vi "image LPF-cluster.vi"(1 "image lpf":cluster{"cutoff ":dbl, "lpf":bool, "order":i32}={"cutoff "=0.0, "lpf"=FALSE, "order"=2}, 2 "x":dbl=1.0 format="%#_13g", 3 "input":dbl[][](array[numeric])) -> (0 "output":dbl[][](array[numeric]))   [LabVIEW 2018]
uses:
  <vilib>/Analysis/3filter.llb/Filter Passband Type.ctl
  <vilib>/Analysis/3filter.llb/Butterworth Filter (DBL).vi
  <vilib>/Analysis/NI_AALBase.lvlib
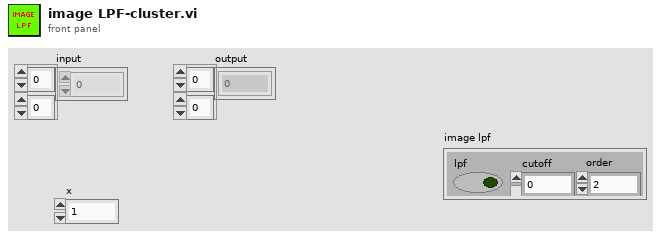
[diagram p1: front panel]
types:
  T1 = typedef "NI_AALBase.lvlib/Filter Passband Type.ctl" = enum32{"Lowpass", "Highpass", "Bandpass", "Bandstop"}
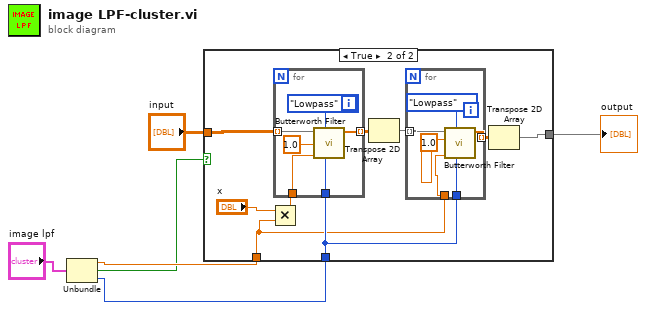
[diagram p0: block diagram]
diagram:
  n1 = Unbundle("image lpf") -> ("cutoff"=w3:dbl, "lpf"=w2:bool, "order"=w1:i32)
  n2 = case shown="True" w2 {
    tunnel: [w7 w16] -> w6
    tunnel: "input" -> [w7 w12]
    tunnel: w1 -> [_ w11]
    tunnel: w3 -> [_ w10]
    frame False {
    }
    frame True {
      n3 = Multiply(x="x", y=w10) -> (x*y=w9:dbl)
      n4 = for {
        tunnel: w12 -> [w26] mode=indexing
        tunnel: [w25] -> w14 mode=indexing
        tunnel: w9 -> [w24]
        tunnel: w11 -> [w23]
        n5 = call-poly <vilib>:"Butterworth Filter.vi"("order"=w23, "filter type"=Filter_Passband_Type."Lowpass", "low cutoff freq: fl"=w24, "sampling freq: fs"=1.0, "X"=w26) -> ("Filtered X"=w25:dbl[])  [unwired: 3 in, 1 out]
      }
      n6 = Transpose 2D Array(2D array=w14) -> (transposed array=w13:dbl[][])
      n7 = for {
        tunnel: w13 -> [w20] mode=indexing
        tunnel: [w19] -> w15 mode=indexing
        tunnel: w10 -> [w18]
        tunnel: w11 -> [w17]
        n8 = call-poly <vilib>:"Butterworth Filter.vi"("order"=w17, "filter type"=Filter_Passband_Type."Lowpass", "low cutoff freq: fl"=w18, "sampling freq: fs"=1.0, "X"=w20) -> ("Filtered X"=w19:dbl[])  [unwired: 3 in, 1 out]
      }
      n9 = Transpose 2D Array(2D array=w15) -> (transposed array=w16:dbl[][])
    }
  }
  "output" <- w6
